vi "Lab4.vi"() -> ()   [LabVIEW 2015]
uses:
  <vilib>/measure/NI_MABase.lvlib
panel:
  out "Waveform Graph":waveform(dbl)(graph)
  out "OFF":bool
  out "c":bool
  out "b":bool
  out "a":bool
  in  "C":bool
  in  "B":bool
  in  "A":bool
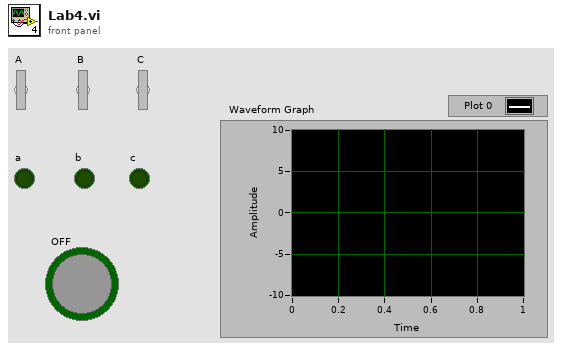
[diagram p1: front panel]
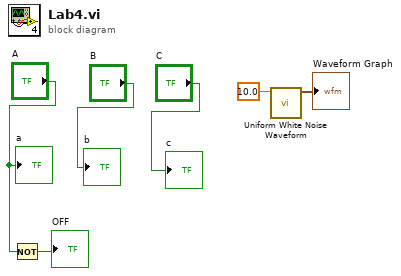
[diagram p0: block diagram]
diagram:
  n1 = Not(x="A") -> (.not. x?=→"OFF":bool)
  n2 = call <vilib>:"Uniform White Noise Waveform.vi"("amplitude"=10.0) -> ("signal out"=→"Waveform Graph":waveform(dbl))  [unwired: 9 in, 1 out]
  "a" <- "A"
  "b" <- "B"
  "c" <- "C"
